vi "KickToSkill_v2.vi"(0 "object in":refnum<class "PassSkill.lvclass">, 5 "error in (no error)":errorcluster) -> (14 "object out":refnum<class "PassSkill.lvclass">, 19 "error out":errorcluster)   [LabVIEW 2023, in "PassSkill.lvclass"]
uses:
  PassSkill.lvclass
  KickToSkill_v2_class/KickToSkill_v2.lvclass
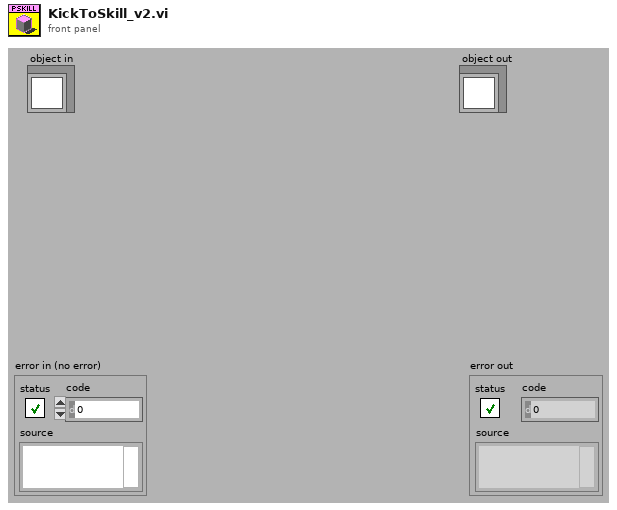
[diagram p1: front panel]
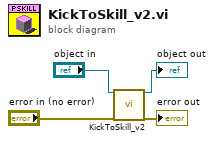
[diagram p0: block diagram]
diagram:
  n1 = call-parent "KickToSkill_v2.vi"("object in"="object in", "error in (no error)"="error in (no error)") -> ("object out"=→"object out":refnum<class "PassSkill.lvclass">, "error out"=→"error out":errorcluster)  [unwired: 16 in]
